vi "ZNB calibration.vi"() -> ()   [LabVIEW 2015]
uses:
  <vilib>/express/express arith-compare/Formula/XNode/ExpressFormulaBlockNode.xnode
  <instrlib>/Rohde&Schwarz Vector Network Analyzer/Rohde&Schwarz Vector Network Analyzer.lvlib
panel:
  in  "VNA's port(s) used for the MI measurements":string(combo)="S11"
  in  "Averaging mode:\n0 - Auto\n1 - Reduce noise\n2 - Flatten noise":i32
  in  "Averaging (ON/OFF)":bool
  in  "Number of averages (>1)":i32
  in  "Filter selectivity (0 - Normal, 1 - High)":i32
  in  "Number of frequency points":i32=5000
  in  "IF Bandwidth (Hz, k - kHz)":dbl=1000.0
  in  "Power (dBm)":dbl
  in  "Stop frequency (k - kHZ, M - MHz, G - GHz)":dbl=20000000000.0
  in  "Start frequency (k - kHz, M - MHz, G - GHz)":dbl=100000.0
  in  "VNA's connection":refnum<visa-resource-name>="ZNB20"
  # "This program prepares a ZNB VNA for the full 2-port manual calibration (TOSM or SOLT). Choose the parameters you need. For the calibration, it is recommended to choose a small IFBW, say 10 KHz, or even 1 kHz. But too small IFBW will result in a very slow sweep.\n\n*****************************************\nDmitriy Makhnovskiy@Hangzhou July 2017\nSensing Materials Technology Ltd, UK\nE-mail: contact@sensmattech.co.uk"
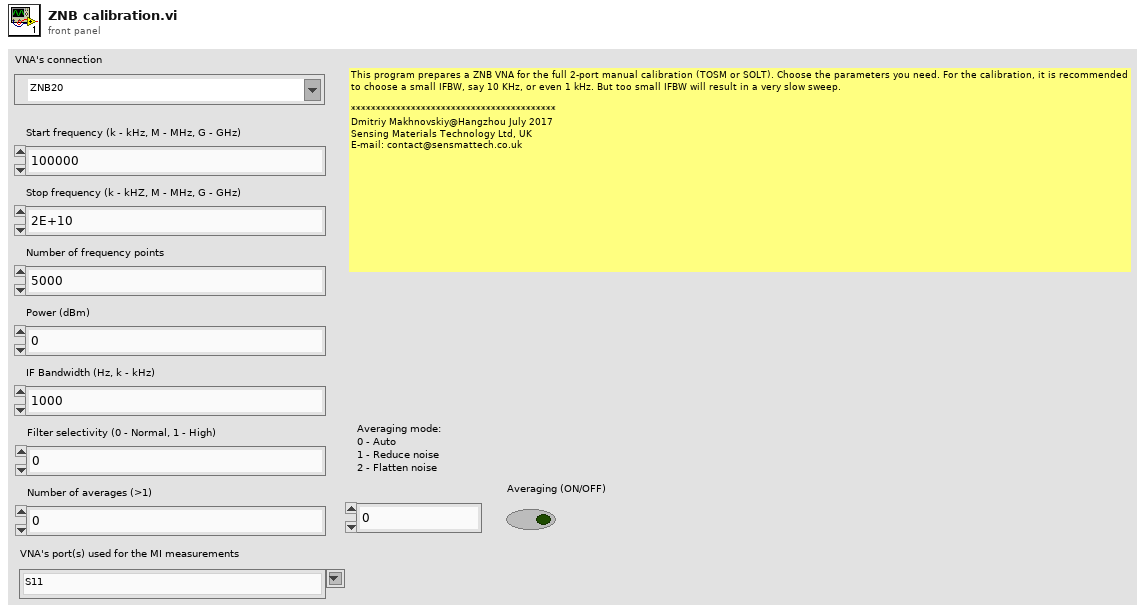
[diagram p1: front panel]
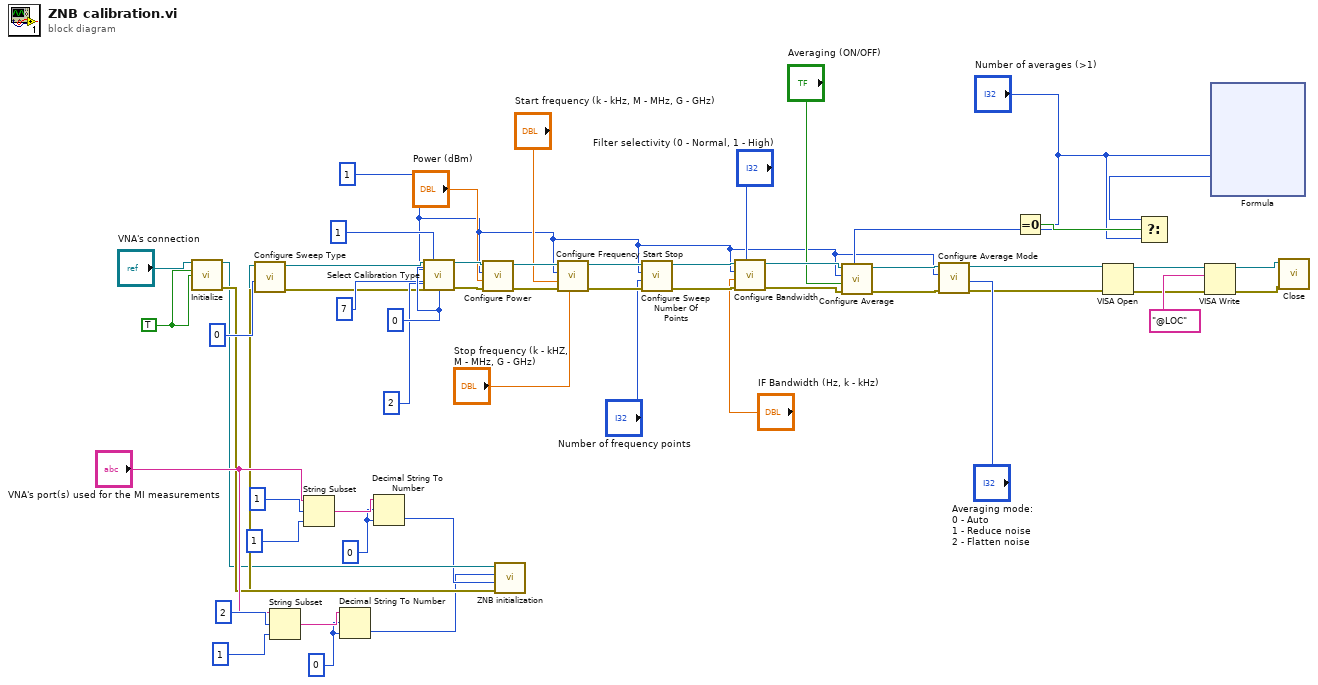
[diagram p0: block diagram]
diagram:
  w1 = 1
  w9 = 0
  w13 = 0
  w54 = 0
  w55 = TRUE
  n1 = call <instrlib>:"Initialize.vi"("VISA resource name"="VNA's connection", "ID Query (T: Check)"=w55, "Reset (T: Reset)"=w55) -> ("VISA resource name out"=w5:refnum<visa-resource-name>, "error out"=w7:errorcluster)  [unwired: 11 in]
  n2 = String Subset(string="VNA's port(s) used for the MI measurements", offset (0)=2, length (rest)=1) -> (substring=w10:string)
  n3 = String Subset(string="VNA's port(s) used for the MI measurements", offset (0)=1, length (rest)=1) -> (substring=w14:string)
  n4 = Decimal String To Number(string=w10, offset=w9, default (0L)=w9) -> (number=w2:i32)  [unwired: 1 out]
  n5 = Decimal String To Number(string=w14, offset=w13, default (0L)=w13) -> (number=w3:i32)  [unwired: 1 out]
  n6 = call "ZNB initialization.vi"("error in (no error)"=w7, "Output port"=w3, "Input port"=w2, "VISA resource name"=w5) -> ("error out"=w6:errorcluster, "VISA resource name out"=w4:refnum<visa-resource-name>)  [unwired: 6 in]
  n7 = call <instrlib>:"Configure Sweep Type.vi"("error in (no error)"=w6, "Sweep Type (Power)"=0, "VISA resource name"=w4) -> ("error out"=w28:errorcluster, "VISA resource name out"=w29:refnum<visa-resource-name>)  [unwired: 7 in]
  n8 = call <instrlib>:"Select Calibration Type.vi"("VISA resource name"=w29, "Port 1 (1)"=1, "Port 3 (1)"=w54, "Channel (1)"=w1, "Parameters (One-port Normalization (reflection, open standard))"=7, "error in (no error)"=w28, "Port 2 (1)"=2, "Port 4 (1)"=w54) -> ("VISA resource name out"=w53:refnum<visa-resource-name>, "error out"=w52:errorcluster)  [unwired: 6 in]
  n9 = call <instrlib>:"Configure Power.vi"("error in (no error)"=w52, "Power (-10.0)"="Power (dBm)", "Channel (1)"=w1, "VISA resource name"=w53) -> ("error out"=w49:errorcluster, "VISA resource name out"=w50:refnum<visa-resource-name>)  [unwired: 6 in]
  n10 = call <instrlib>:"Configure Frequency Start Stop.vi"("Stop Frequency (4.0e9)"="Stop frequency (k - kHZ, M - MHz, G - GHz)", "error in (no error)"=w49, "Start Frequency (300.0e3)"="Start frequency (k - kHz, M - MHz, G - GHz)", "Channel (1)"=w1, "VISA resource name"=w50) -> ("error out"=w45:errorcluster, "VISA resource name out"=w46:refnum<visa-resource-name>)  [unwired: 5 in]
  n11 = call <instrlib>:"Configure Sweep Number Of Points.vi"("error in (no error)"=w45, "Number Of Points (201)"="Number of frequency points", "Channel (1)"=w1, "VISA resource name"=w46) -> ("error out"=w42:errorcluster, "VISA resource name out"=w43:refnum<visa-resource-name>)  [unwired: 6 in]
  n12 = call <instrlib>:"Configure Bandwidth.vi"("Filter Selectivity (Normal)"="Filter selectivity (0 - Normal, 1 - High)", "error in (no error)"=w42, "Bandwidth (10.0e3)"="IF Bandwidth (Hz, k - kHz)", "Channel (1)"=w1, "VISA resource name"=w43) -> ("error out"=w36:errorcluster, "VISA resource name out"=w37:refnum<visa-resource-name>)  [unwired: 5 in]
  n13 = Equal To 0?(x="Number of averages (>1)") -> (x = 0?=w26:bool)
  n14 = xnode "Formula"("X1"="Number of averages (>1)") -> ("Result"=w23:i32)  [unwired: 1 in, 1 out]
  n15 = Select(t=w23, s=w26, f="Number of averages (>1)") -> (s? t:f=w24:i32)
  n16 = call <instrlib>:"Configure Average.vi"("Average Factor (10)"=w24, "error in (no error)"=w36, "Average State (Off)"="Averaging (ON/OFF)", "Channel (1)"=w1, "VISA resource name"=w37) -> ("error out"=w33:errorcluster, "VISA resource name out"=w34:refnum<visa-resource-name>)  [unwired: 5 in]
  n17 = call <instrlib>:"Configure Average Mode.vi"("error in (no error)"=w33, "Mode (Auto)"="Averaging mode:\n0 - Auto\n1 - Reduce noise\n2 - Flatten noise", "Channel (1)"=w1, "VISA resource name"=w34) -> ("error out"=w17:errorcluster, "VISA resource name out"=w18:refnum<visa-resource-name>)  [unwired: 6 in]
  n18 = VISA Open(error in (no error)=w17, VISA resource name=w18) -> (VISA resource name=w20:refnum<visa-resource-name>, error out=w19:errorcluster)  [unwired: 3 in]
  n19 = VISA Write(VISA resource name=w20, write buffer="@LOC", error in (no error)=w19) -> (VISA resource name out=w22:refnum<visa-resource-name>, error out=w21:errorcluster)  [unwired: 1 out]
  n20 = call <instrlib>:"Close.vi"("error in (no error)"=w21, "VISA resource name"=w22) -> ()  [unwired: 9 in, 1 out]
